vi "Configure I2S settings.vi"(8 "error in (no error)":errorcluster, 11 "Measurement Configuration":T2={"Band start"=20.0, "Band stop"=20000.0, "Weighting filter"=0, "Full scale range"=3.16, "Analog source resource name"="", "Frequency"=1000.0, "Amplitude"=1.0, "Protocol capture resource name"="PXI1Slot7\\I2Si 0", "Protocol capture channel"="", "Clock rate"=12288000, "Number of words"=19200, "Sensitivity"=0.34762, "JSONFile"=""}) -> (0 "error out":errorcluster, 3 "PCM input task out":T1)   [LabVIEW 2021, in "audio_acMeasurement.lvlib"]
uses:
  audio_acMeasurement.lvlib
  Measurement Configuration.ctl
  <vilib>/PDM Acquisition Toolkit/host/Classes/Tasks/PCM Input/Controls/DVR PCM Input Task.ctl
  <vilib>/PDM Acquisition Toolkit/host/Classes/Tasks/PCM Input/PCM Input Task.lvclass
  <vilib>/PDM Acquisition Toolkit/host/Classes/Tasks/PDM Tasks/Controls/Acquisition Mode.ctl
  <vilib>/PDM Acquisition Toolkit/host/Classes/Session/Controls/Logic Levels.ctl
  <vilib>/PDM Acquisition Toolkit/host/API/Public/Create Tasks/Create PCM Input Task.vi
  <vilib>/PDM Acquisition Toolkit/host/API/Public/Configure/Timing/Configure Timing - PCM Input Slave.vi
  <vilib>/PDM Acquisition Toolkit/host/API/PDM Acquisition Toolkit.lvlib
  <vilib>/PDM Acquisition Toolkit/host/Classes/Tasks/PDM Tasks/PDM Task.lvclass
  <vilib>/PDM Acquisition Toolkit/host/Classes/Session/DecoderSession.lvclass
  <vilib>/PDM Acquisition Toolkit/host/API/Public/Configure/PDM Channel/Configure Microphone Sensitivity FSPA - PCM Input Task.vi
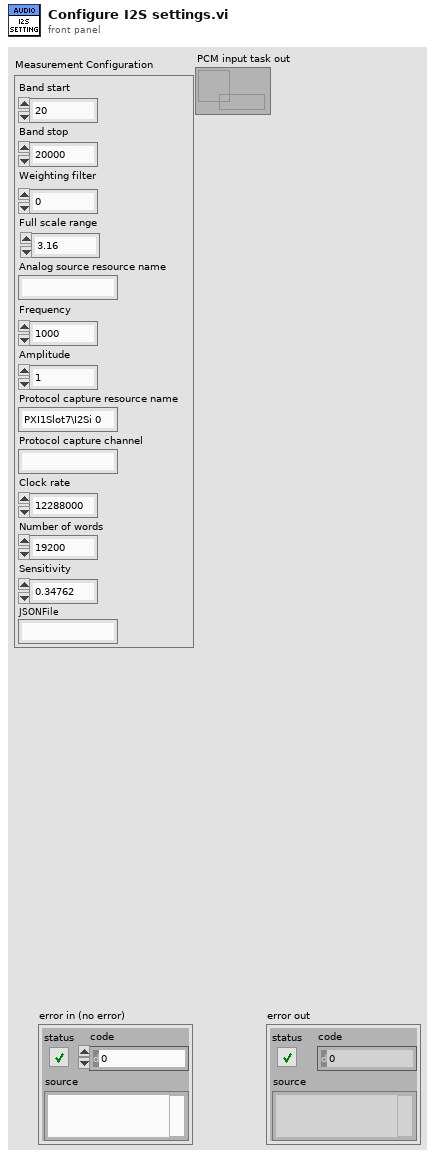
[diagram p1: front panel]
types:
  T1 = typedef "PDM Acquisition Class Library.lvlib/PCM Input Task.lvclass/DVR PCM Input Task.ctl" = refnum<data-value>
  T2 = typedef "audio_acMeasurement.lvlib/Measurement Configuration.ctl" = cluster{"Band start":dbl, "Band stop":dbl, "Weighting filter":u16, "Full scale range":dbl, "Analog source resource name":string, "Frequency":dbl, "Amplitude":dbl, "Protocol capture resource name":string, "Protocol capture channel":string, "Clock rate":u32, "Number of words":u32, "Sensitivity":dbl, "JSONFile":string}
  T3 = cluster{"PCM Data Configuration":cluster{"Frame_Sync_Edge_for_Channel 0":i32, "Channel_Count_Per_Frame":i32, "Channel_Length":i32, "Bit_Depth":i32, "Channel_0_Offset":i32, "Endianness":i32, "Data_Justification":i32}, "Frame Sync Clock Control":cluster{"Frame_Length":i32, "Frame_Sync_Pulse_Width":i32, "Bit_Clock_Edge_Sync":i32}}
  T4 = enum16{"open", "replace", "create", "open or create", "replace or create", "replace or create with confirmation"}
  T5 = typedef "PDM Acquisition Class Library.lvlib/DecoderSession.lvclass/Logic Levels.ctl" = enum16{"3.3 V", "1.8 V", "1.2 V"}
  T6 = typedef "PDM Acquisition Class Library.lvlib/PDM Task.lvclass/Acquisition Mode.ctl" = enum16{"Finite", "Continuous"}
  T7 = cluster{"Frame_Sync_Edge_for_Channel 0":i32, "Channel_Count_Per_Frame":i32, "Channel_Length":i32, "Bit_Depth":i32, "Channel_0_Offset":i32, "Endianness":i32, "Data_Justification":i32}
  T8 = cluster{"Frame_Length":i32, "Frame_Sync_Pulse_Width":i32, "Bit_Clock_Edge_Sync":i32}
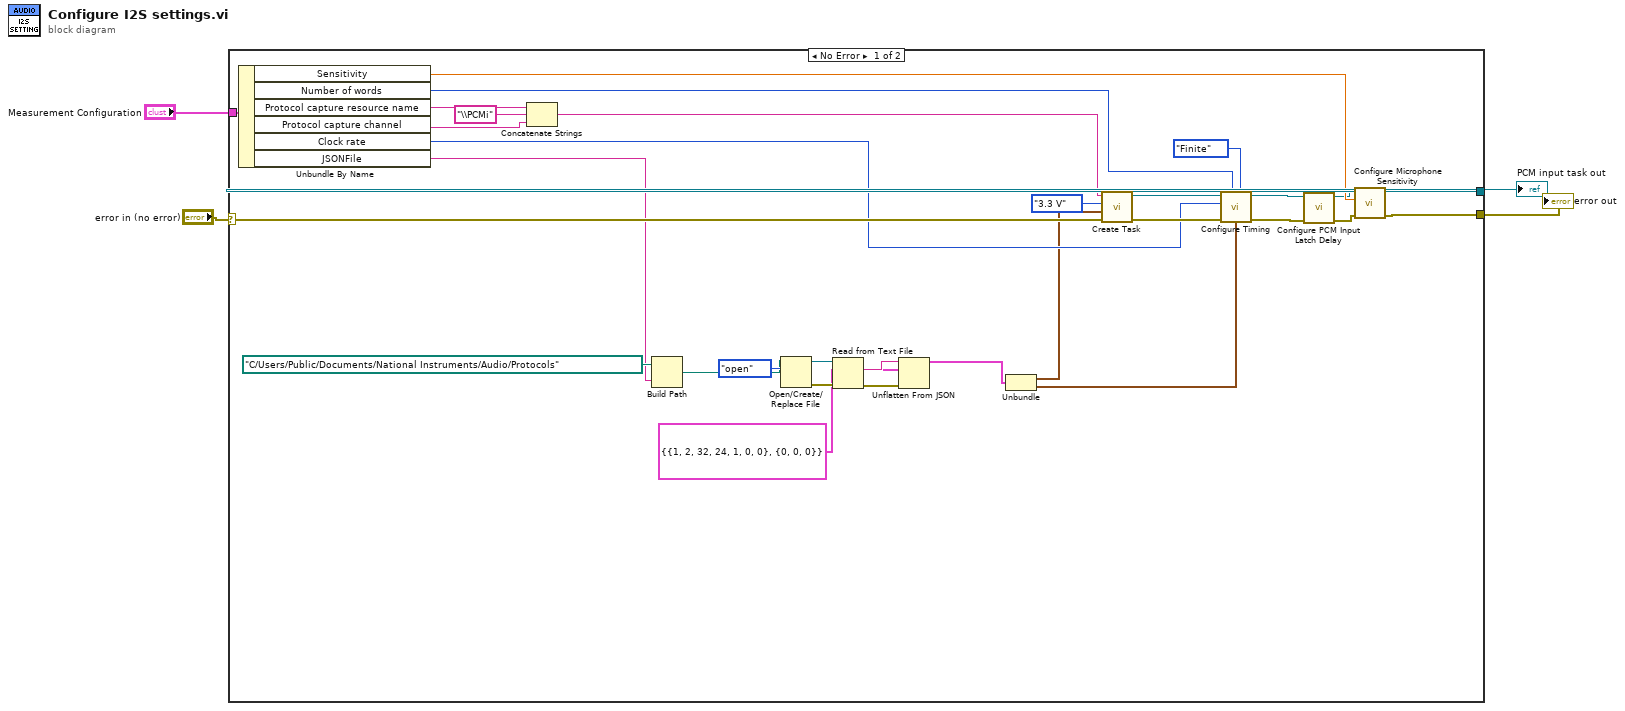
[diagram p0: block diagram]
diagram:
  n1 = case shown="No Error" "error in (no error)" {
    selector: "error in (no error)" -> [w30 w36]
    tunnel: [w17 w36] -> w4
    tunnel: "Measurement Configuration" -> [w34 _]
    tunnel: [w18 _] -> w1
    frame No Error {
      n2 = Unbundle By Name(w34) -> ("Sensitivity"=w21:dbl, "Number of words"=w35:u32, "Protocol capture resource name"=w27:string, "Protocol capture channel"=w25:string, "Clock rate"=w28:u32, "JSONFile"=w5:string)
      n3 = Concatenate Strings(w27, "\\PCMi" ("element"), w25) -> (w24:string)
      n4 = Build Path(base path=path "C:/Users/Public/Documents/National Instruments/Audio/Protocols", name or relative path=w5) -> (appended path=w10:path)
      n5 = Open/Create/Replace File(file path (use dialog)=w10, operation (0:open)=T4."open") -> (refnum out=w14:refnum<file>, error out=w12:errorcluster)  [unwired: 4 in, 1 out]
      n6 = Read from Text File(file (use dialog)=w14, error in=w12) -> (text=w15:string, error out=w13:errorcluster)  [unwired: 2 in, 2 out]
      n7 = Unflatten From JSON(JSON string=w15, type and defaults=T3 {"PCM Data Configuration"={"Frame_Sync_Edge_for_Channel 0"=1, "Channel_Count_Per_Frame"=2, "Channel_Length"=32, "Bit_Depth"=24, "Channel_0_Offset"=1, "Endianness"=0, "Data_Justification"=0}, "Frame Sync Clock Control"={"Frame_Length"=0, "Frame_Sync_Pulse_Width"=0, "Bit_Clock_Edge_Sync"=0}}, error in (no error)=w13) -> (value=w9:T3)  [unwired: 4 in, 1 out]
      n8 = Unbundle(w9) -> ("PCM Data Configuration"=w6:T7, "Frame Sync Clock Control"=w7:T8)
      n9 = call-poly <vilib>:"Create Task.vi"("error in"=w30, "PCM data configuration"=w6, "logic level"=Logic_Levels."3.3 V", "channel list"=w24) -> ("error out"=w32:errorcluster, "PCM input task out"=w33:T1)  [unwired: 6 in]
      n10 = call-poly <vilib>:"Configure Timing.vi"("acquisition mode"=Acquisition_Mode."Finite", "Frame Sync Clock Control"=w7, "number of words per channel"=w35, "error in"=w32, "Bit Clock rate"=w28, "PCM input task in"=w33) -> ("error out"=w22:errorcluster, "PCM input task out"=w23:T1)  [unwired: 4 in]
      n11 = call <vilib>:"Configure PCM Input Latch Delay.vi"("error in"=w22, "PCM input task in"=w23) -> ("error out"=w19:errorcluster, "PCM input task out"=w20:T1)  [unwired: 7 in, 1 out]
      n12 = call-poly <vilib>:"Configure Microphone Sensitivity.vi"("error in"=w19, "microphone sensitivity (FS/Pa)"=w21, "PCM input task in"=w20) -> ("error out"=w17:errorcluster, "PCM input task out"=w18:T1)  [unwired: 7 in]
    }
    frame Error {
    }
  }
  "error out" <- w4
  "PCM input task out" <- w1
